vi "Set 2D Ramp Rates_manual_ramp_brasse_v1.vi"(0 "Y-Axis Communications Config":T1={"GPIB address"=22, "GPIB bus"=0, "connection ID"=refnum, "IP"="192.168.2.200", "Active Comm Interface"=0, "Serial Port"="", "Programmer Type"=0} {"Programmer Type" items=["Model 430", "Model 420"]; "Active Comm Interface" items=["TCP/IP (Model 430 Only)", "RS232", "IEEE488"]}, 1 "Y-Axis Field (kG)":dbl format="%.3f", 2 "Y-Axis ramp?":bool=TRUE, 3 "Next Y-Axis Field (kG)":dbl format="%.3f", 4 "Z-Axis Communications Config":T1={"GPIB address"=22, "GPIB bus"=0, "connection ID"=refnum, "IP"="192.168.2.200", "Active Comm Interface"=0, "Serial Port"="", "Programmer Type"=0} {"Programmer Type" items=["Model 430", "Model 420"]; "Active Comm Interface" items=["TCP/IP (Model 430 Only)", "RS232", "IEEE488"]}, 5 "Z-Axis Field (kG)":dbl format="%.3f", 6 "User defined Ramp Rate (T/min)":bool, 7 "Next Z-Axis Field (kG)":dbl format="%.3f", 8 "Max Ramp Rate - Y Axis (A/s)":dbl format="%.3f", 9 "Max Ramp Rate - Z Axis (A/s)":dbl format="%.3f", 10 "User defined Ramp Rate - Z Axis (kG/s)":dbl format="%.3f", 11 "error in":T2, 12 "User defined Ramp Rate Y-Axis (kG/s)":dbl format="%.3f", 13 "Z-Axis ramp?":bool=TRUE) -> (15 "Y-Axis Ramp Rate (T/min)":dbl format="%.3f", 17 "Z-Axis Ramp Rate (T/min)":dbl format="%.3f", 18 "error out":T2)   [LabVIEW 2009]
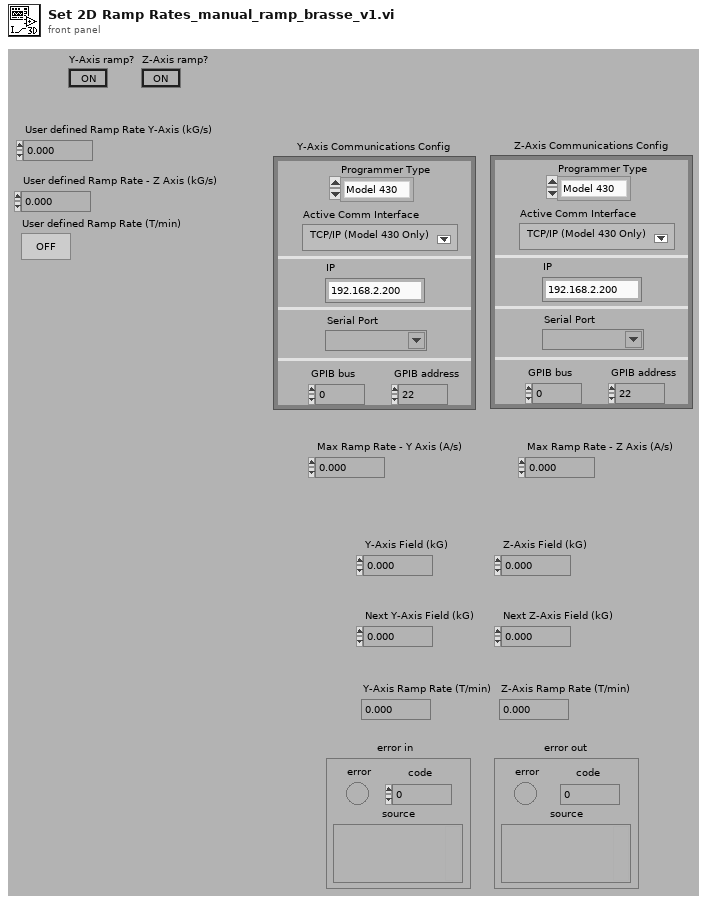
[diagram p1: front panel]
types:
  T1 = cluster{"GPIB address":i16, "GPIB bus":i16, "connection ID":refnum<k5>, "IP":string, "Active Comm Interface":u16, "Serial Port":refnum<visa-resource-name>, "Programmer Type":u16}
  T2 = cluster{"error":bool, "code":i32, "source":string}
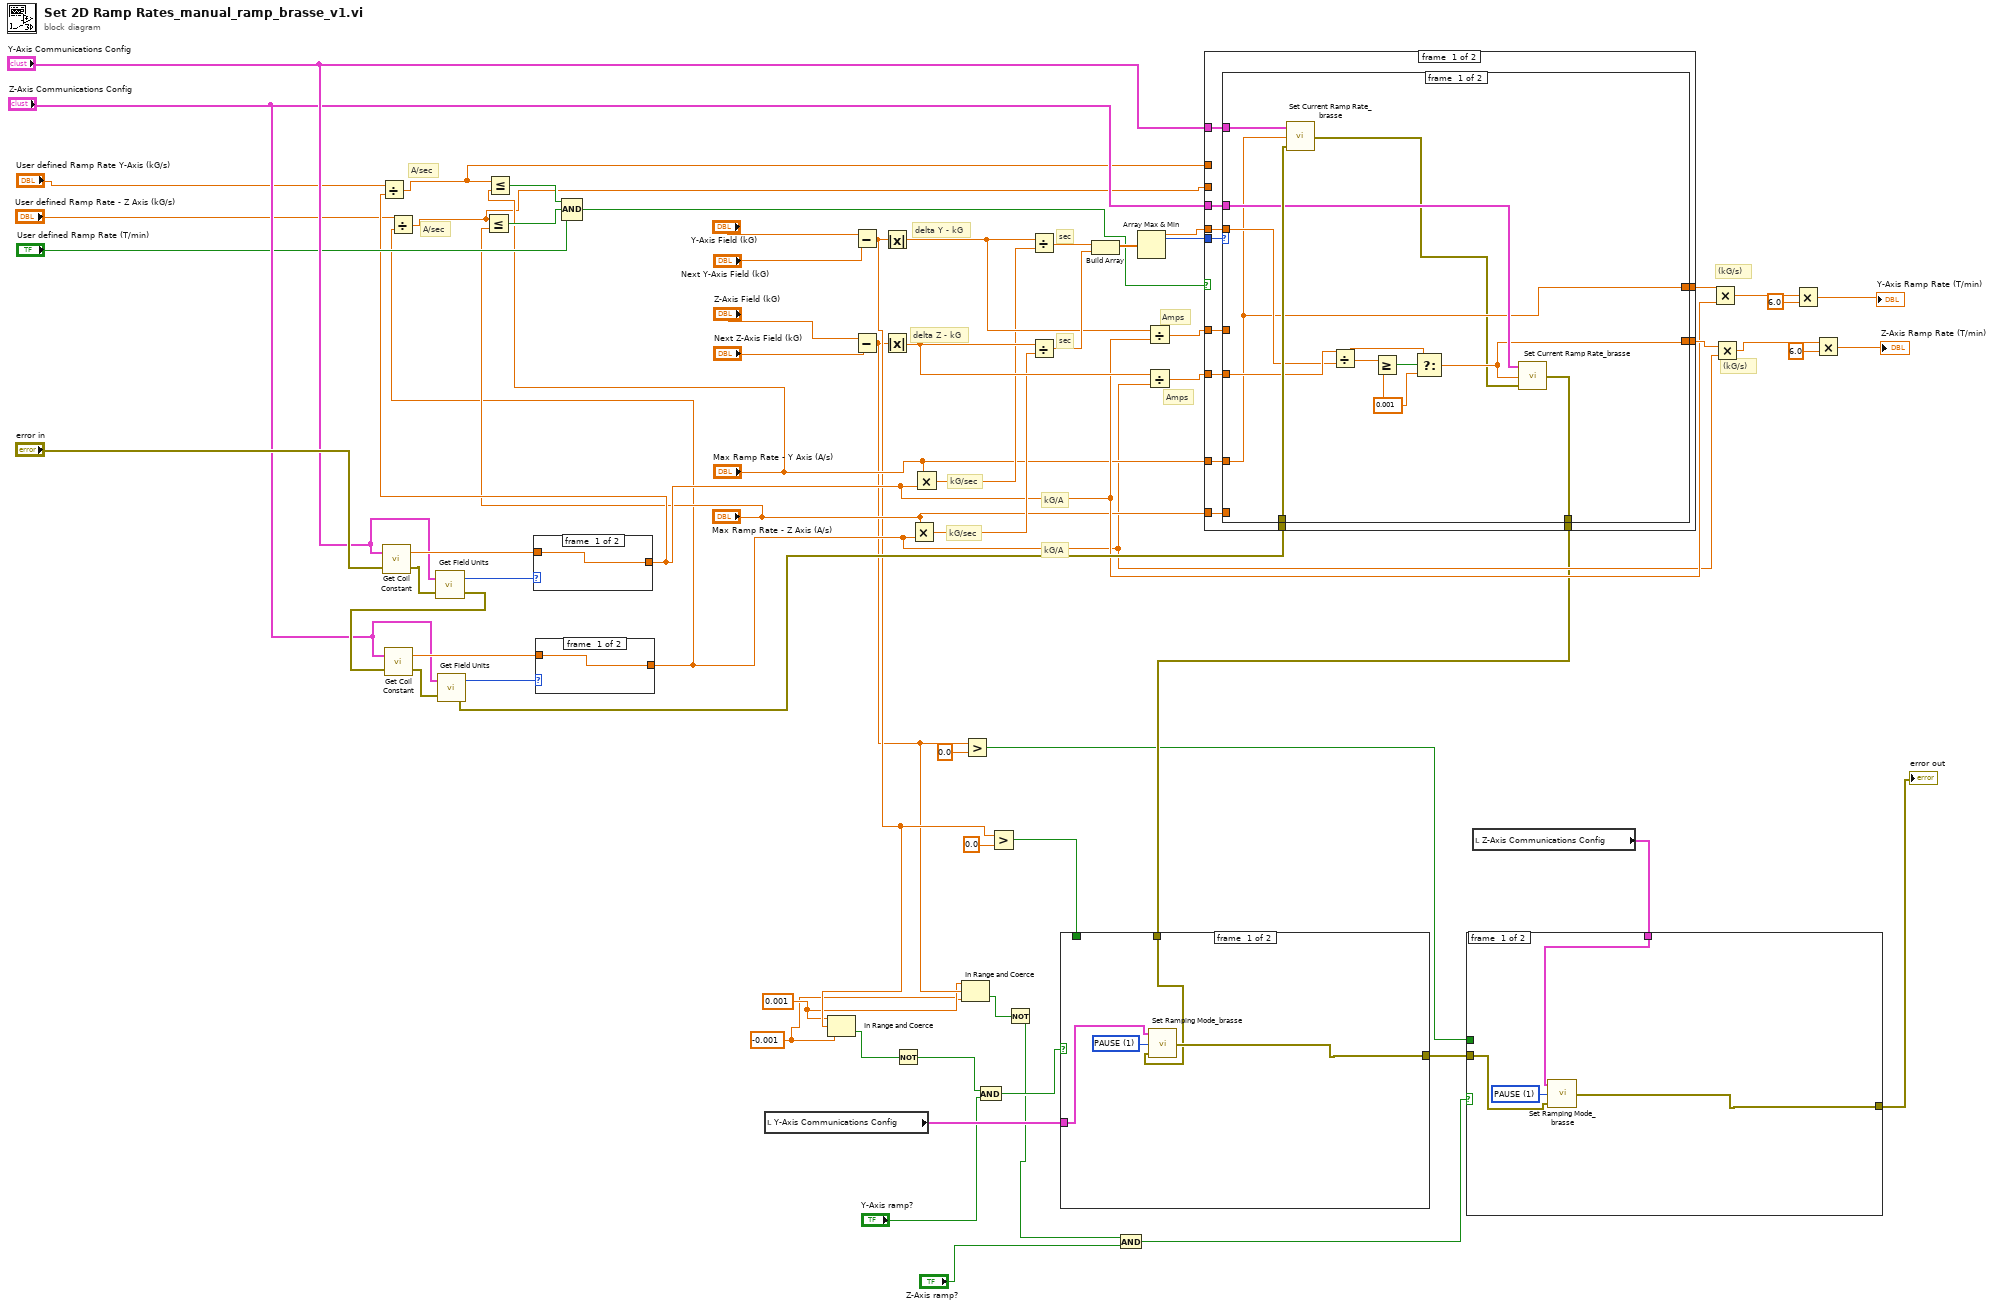
[diagram p0: block diagram]
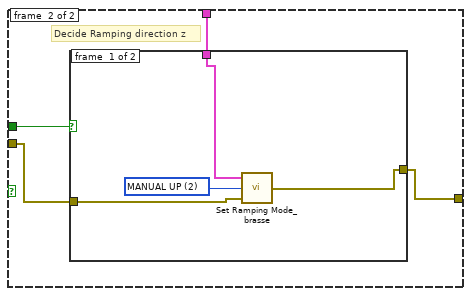
[diagram p2: hidden frame]
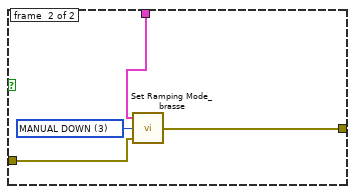
[diagram p3: hidden frame]
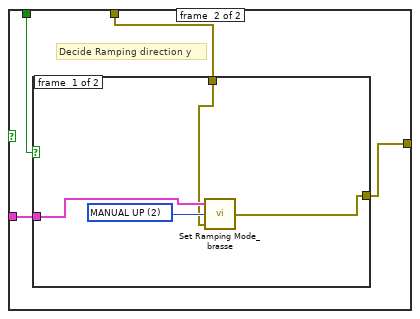
[diagram p4: hidden frame]
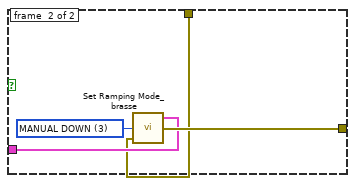
[diagram p5: hidden frame]
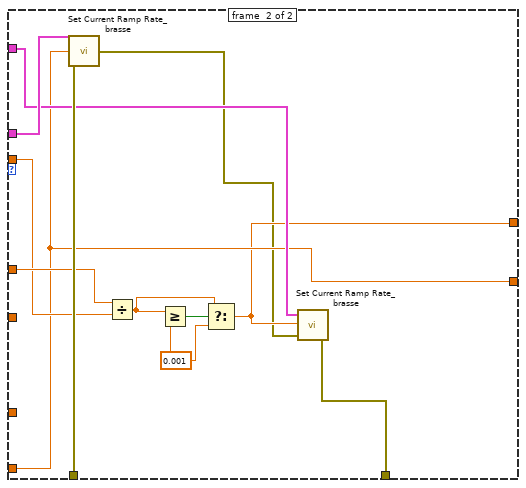
[diagram p6: hidden frame]
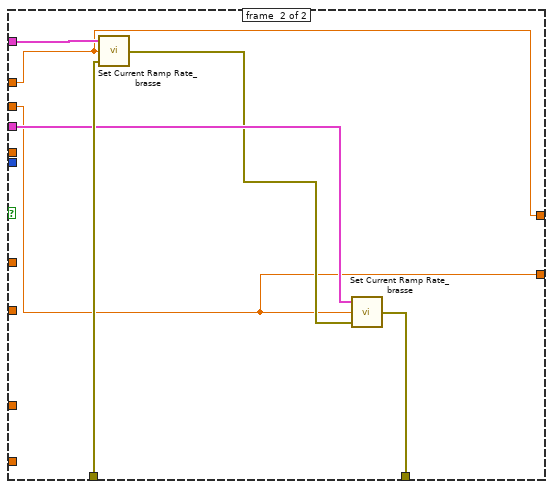
[diagram p7: hidden frame]
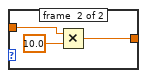
[diagram p8: hidden frame]
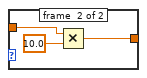
[diagram p9: hidden frame]
diagram:
  w3 = -0.001 ("lower limit")
  w4 = 0.001 ("upper limit")
  # "(kG/s)"
  # "(kG/s)"
  # "A/sec"
  # "A/sec"
  # "Amps"
  # "Amps"
  # "kG/A"
  # "kG/A"
  # "kG/sec"
  # "kG/sec"
  # "delta Z - kG"
  # "delta Y - kG"
  # "sec"
  # "sec"
  n1 = call <userlib>:"Get Coil Constant.vi"("error in"="error in", "Communications Config"="Y-Axis Communications Config") -> ("error out"=w50:T2, "Coil Constant"=w51:dbl)
  n2 = call <userlib>:"Get Field Units.vi"("error in"=w50, "Communications Config"="Y-Axis Communications Config") -> ("error out"=w46:T2, "Field Units"=w52:enum16{"kg", "t"})
  n3 = call <userlib>:"Get Coil Constant.vi"("error in"=w46, "Communications Config"="Z-Axis Communications Config") -> ("error out"=w47:T2, "Coil Constant"=w48:dbl)
  n4 = call <userlib>:"Get Field Units.vi"("error in"=w47, "Communications Config"="Z-Axis Communications Config") -> ("error out"=w45:T2, "Field Units"=w49:enum16{"kg", "t"})
  n5 = case shown="\"t\"" w52 {
    tunnel: w51 -> [w68 w70]
    tunnel: [w68 w69] -> w33
    frame #0 {
    }
    frame #1 {
      n6 = Multiply(x=w70, y=10.0) -> (x*y=w69:dbl)
    }
  }
  n7 = Divide(x="User defined Ramp Rate Y-Axis (kG/s)", y=w33) -> (x/y=w34:dbl)
  n8 = Less Or Equal?(x=w34, y="Max Ramp Rate - Y Axis (A/s)") -> (x <= y?=w39:bool)
  n9 = case shown="\"t\"" w49 {
    tunnel: w48 -> [w72 w74]
    tunnel: [w72 w73] -> w29
    frame #0 {
    }
    frame #1 {
      n10 = Multiply(x=w74, y=10.0) -> (x*y=w73:dbl)
    }
  }
  n11 = Divide(x="User defined Ramp Rate - Z Axis (kG/s)", y=w29) -> (x/y=w28:dbl)
  n12 = Less Or Equal?(x=w28, y="Max Ramp Rate - Z Axis (A/s)") -> (x <= y?=w38:bool)
  n13 = Compound Arithmetic op=AND(w39, w38, "User defined Ramp Rate (T/min)") -> (w36:bool)
  n14 = local read "Y-Axis Communications Config"() -> (w17:T1)
  n15 = Subtract(x="Y-Axis Field (kG)", y="Next Y-Axis Field (kG)") -> (x-y=w8:dbl)
  n16 = In Range and Coerce(upper limit=w4, x=w8, lower limit=w3) -> (In Range?=w7:bool)  [unwired: 1 out]
  n17 = Subtract(x="Z-Axis Field (kG)", y="Next Z-Axis Field (kG)") -> (x-y=w5:dbl)
  n18 = Absolute Value(x=w8) -> (abs(x)=w59:dbl)
  n19 = Absolute Value(x=w5) -> (abs(x)=w58:dbl)
  n20 = Not(x=w7) -> (.not. x?=w6:bool)
  n21 = Multiply(x="Max Ramp Rate - Z Axis (A/s)", y=w29) -> (x*y=w41:dbl)
  n22 = Multiply(x="Max Ramp Rate - Y Axis (A/s)", y=w33) -> (x*y=w40:dbl)
  n23 = In Range and Coerce(upper limit=w4, x=w5, lower limit=w3) -> (In Range?=w2:bool)  [unwired: 1 out]
  n24 = Greater?(x=w5, y=0.0) -> (0:w12:bool)
  n25 = And(x=w6, y="Y-Axis ramp?") -> (x .and. y?=w14:bool)
  n26 = Greater?(x=w8, y=0.0) -> (0:w16:bool)
  n27 = Not(x=w2) -> (.not. x?=w1:bool)
  n28 = Divide(x=w59, y=w40) -> (x/y=w67:dbl)
  n29 = Divide(x=w58, y=w41) -> (x/y=w66:dbl)
  n30 = Build Array(w67, w66) -> (w60:dbl[])
  n31 = And(x=w1, y="Z-Axis ramp?") -> (x .and. y?=w9:bool)
  n32 = Array Max & Min(array=w60) -> (max value=w57:dbl, max index (indices)=w61:i32)  [unwired: 2 out]
  n33 = Divide(x=w59, y=w33) -> (x/y=w56:dbl)
  n34 = Divide(x=w58, y=w29) -> (x/y=w55:dbl)
  n35 = case shown="False" w36 {
    tunnel: w61 -> [w87 _]
    tunnel: w57 -> [w86 _]
    tunnel: w56 -> [w85 _]
    tunnel: w55 -> [w84 _]
    tunnel: [w83 w113] -> w54
    tunnel: [w82 w112] -> w53
    tunnel: w45 -> [w81 w118]
    tunnel: "Max Ramp Rate - Y Axis (A/s)" -> [w80 _]
    tunnel: "Max Ramp Rate - Z Axis (A/s)" -> [w79 _]
    tunnel: [w78 w117] -> w13
    tunnel: "Y-Axis Communications Config" -> [w77 w116]
    tunnel: "Z-Axis Communications Config" -> [w76 w115]
    tunnel: w34 -> [_ w113]
    tunnel: w28 -> [_ w112]
    frame #0 {
      n36 = case shown="1" w87 {
        tunnel: w81 -> [w98 w110]
        tunnel: w86 -> [w96 w108]
        tunnel: w85 -> [_ w109]
        tunnel: w77 -> [w99 w107]
        tunnel: w84 -> [w97 _]
        tunnel: w76 -> [w95 w111]
        tunnel: [w94 w106] -> w78
        tunnel: [w93 w101] -> w83
        tunnel: [w89 w105] -> w82
        tunnel: w80 -> [w93 _]
        tunnel: w79 -> [_ w105]
        frame #0 {
          w92 = 0.001 ("f")
          n37 = call "Set Current Ramp Rate_brasse.vi"("Communications Config"=w99, "Ramp Rate (A/sec)"=w93, "error in"=w98) -> ("error out"=w88:T2)  [unwired: 2 in]
          n38 = Divide(x=w97, y=w96) -> (x/y=w90:dbl)
          n39 = Greater Or Equal?(x=w90, y=w92) -> (x >= y?=w91:bool)
          n40 = Select(t=w90, s=w91, f=w92) -> (s? t:f=w89:dbl)
          n41 = call "Set Current Ramp Rate_brasse.vi"("Communications Config"=w95, "Ramp Rate (A/sec)"=w89, "error in"=w88) -> ("error out"=w94:T2)  [unwired: 2 in]
        }
        frame #1 {
          w104 = 0.001 ("f")
          n42 = call "Set Current Ramp Rate_brasse.vi"("Communications Config"=w111, "Ramp Rate (A/sec)"=w105, "error in"=w110) -> ("error out"=w100:T2)  [unwired: 2 in]
          n43 = Divide(x=w109, y=w108) -> (x/y=w102:dbl)
          n44 = Greater Or Equal?(x=w102, y=w104) -> (x >= y?=w103:bool)
          n45 = Select(t=w102, s=w103, f=w104) -> (s? t:f=w101:dbl)
          n46 = call "Set Current Ramp Rate_brasse.vi"("Communications Config"=w107, "Ramp Rate (A/sec)"=w101, "error in"=w100) -> ("error out"=w106:T2)  [unwired: 2 in]
        }
      }
    }
    frame #1 {
      n47 = call "Set Current Ramp Rate_brasse.vi"("Communications Config"=w116, "Ramp Rate (A/sec)"=w113, "error in"=w118) -> ("error out"=w114:T2)  [unwired: 2 in]
      n48 = call "Set Current Ramp Rate_brasse.vi"("Communications Config"=w115, "Ramp Rate (A/sec)"=w112, "error in"=w114) -> ("error out"=w117:T2)  [unwired: 2 in]
    }
  }
  n49 = case shown="False" w14 {
    tunnel: [w121 w123] -> w19
    tunnel: w17 -> [w120 w126]
    tunnel: w16 -> [_ w125]
    tunnel: w13 -> [w119 w124]
    frame #0 {
      w122 = u16 1 items=["RAMP", "PAUSE", "MANUAL UP", "MANUAL DOWN", "ZERO"] ("Ramping Mode")
      n50 = call "Set Ramping Mode_brasse.vi"("error in"=w119, "Ramping Mode"=w122, "Communications Config"=w120) -> ("error out"=w121:T2)
    }
    frame #1 {
      # "Decide Ramping direction y"
      n51 = case shown="False" w125 {
        tunnel: [w129 w134] -> w123
        tunnel: w126 -> [w128 w132]
        tunnel: w124 -> [w127 w131]
        frame #0 {
          w130 = u16 2 items=["RAMP", "PAUSE", "MANUAL UP", "MANUAL DOWN", "ZERO"] ("Ramping Mode")
          n52 = call "Set Ramping Mode_brasse.vi"("error in"=w127, "Ramping Mode"=w130, "Communications Config"=w128) -> ("error out"=w129:T2)
        }
        frame #1 {
          w133 = u16 3 items=["RAMP", "PAUSE", "MANUAL UP", "MANUAL DOWN", "ZERO"] ("Ramping Mode")
          n53 = call "Set Ramping Mode_brasse.vi"("error in"=w131, "Ramping Mode"=w133, "Communications Config"=w132) -> ("error out"=w134:T2)
        }
      }
    }
  }
  n54 = local read "Z-Axis Communications Config"() -> (w11:T1)
  n55 = case shown="False" w9 {
    tunnel: [w137 w139] -> w18
    tunnel: w19 -> [w136 w140]
    tunnel: w12 -> [_ w142]
    tunnel: w11 -> [w135 w141]
    frame #0 {
      w138 = u16 1 items=["RAMP", "PAUSE", "MANUAL UP", "MANUAL DOWN", "ZERO"] ("Ramping Mode")
      n56 = call "Set Ramping Mode_brasse.vi"("error in"=w136, "Ramping Mode"=w138, "Communications Config"=w135) -> ("error out"=w137:T2)
    }
    frame #1 {
      # "Decide Ramping direction z"
      n57 = case shown="False" w142 {
        tunnel: [w145 w150] -> w139
        tunnel: w141 -> [w144 w148]
        tunnel: w140 -> [w143 w147]
        frame #0 {
          w146 = u16 2 items=["RAMP", "PAUSE", "MANUAL UP", "MANUAL DOWN", "ZERO"] ("Ramping Mode")
          n58 = call "Set Ramping Mode_brasse.vi"("error in"=w143, "Ramping Mode"=w146, "Communications Config"=w144) -> ("error out"=w145:T2)
        }
        frame #1 {
          w149 = u16 3 items=["RAMP", "PAUSE", "MANUAL UP", "MANUAL DOWN", "ZERO"] ("Ramping Mode")
          n59 = call "Set Ramping Mode_brasse.vi"("error in"=w147, "Ramping Mode"=w149, "Communications Config"=w148) -> ("error out"=w150:T2)
        }
      }
    }
  }
  "error out" <- w18
  n60 = Multiply(x=w54, y=w33) -> (x*y=w24:dbl)
  n61 = Multiply(x=w53, y=w29) -> (x*y=w27:dbl)
  n62 = Multiply(x=w24, y=6.0) -> (x*y=→"Y-Axis Ramp Rate (T/min)":dbl)
  n63 = Multiply(x=w27, y=6.0) -> (x*y=→"Z-Axis Ramp Rate (T/min)":dbl)
